vi "test.vi"() -> ()   [LabVIEW 2019]
uses:
  class/mqtt/mqttTypedef/mqttConnectionMeta.ctl
  class/mqtt/mqttTypedef/mqttQOSlevel.ctl
  class/mqtt/mqttTypedef/mqttSubscribeCluster.ctl
  class/mqtt/mqttTypedef/mqttConnectionStatus.ctl
  class/mqtt/mqttTXqueue/mqttTXdataQueueFunction.ctl
  class/mqtt/mqttConfigFunction.ctl
  class/mqtt/mqttTXqueue/mqttRXsubscriptionEventFunction.ctl
  class/mqtt/mqttTypedef/mqttBroker.ctl
  class/mqtt/mqttTypedef/mqttConnectionFlags.ctl
  class/mqtt/mqttTypedef/mqttWillInformation.ctl
  class/mqtt/mqtt.lvclass
panel:
  out "Ping Success":bool=TRUE
  in  "pingRequest":bool
  out "Numeric":i32
  out "messageID":u16
  out "RX Value":string
  out "RX Topic":string
  in  "includeTimeStamp":bool=TRUE
  in  "disconnect":bool
  out "sessionPresent":bool
  out "connStatus":T1
  in  "connect":bool
  in  "subscriptionInfo":T2[](array[typedef])=[{"Topic"="a/b", "QoS"=enum."At most once"}]
  out "subscribeMessageID":u16 format="%02x"
  out "subscribeSuccess":bool
  out "publishSuccess":bool=TRUE
  out "valueSent":string="14:19:17.238_"
  out "publishMessageID":u16 format="%02x"
  in  "connMeta":T4
  in  "value":string="abc"
  in  "topic":string="a/b"
  in  "quit":bool
  in  "subscribe":bool
  in  "publish":bool
  out "error out":errorcluster
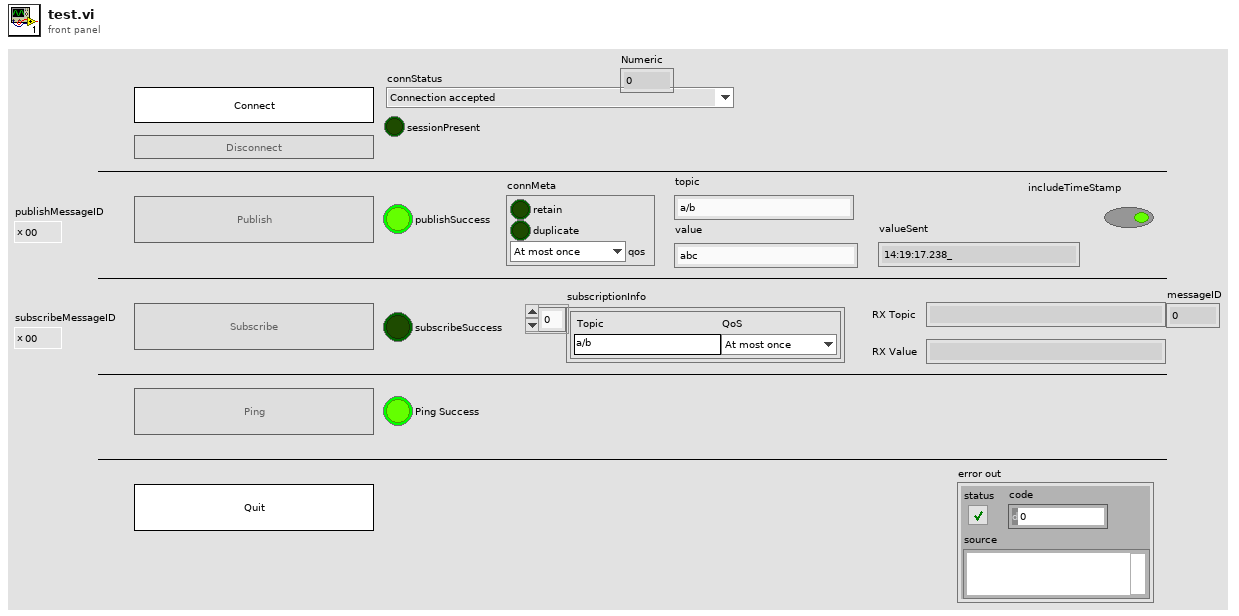
[diagram p1: front panel]
types:
  T1 = typedef "mqttConnectionStatus.ctl" = enum16{"Connection accepted", "Connection refused: unacceptable protocol version", "Connection refused: identifier rejected", "Connection refused: Server unavailable", "Connection refused: bad user name or password", "Connection refused: not authorized"}
  T2 = typedef "mqttSubscribeCluster.ctl" = cluster{"Topic":string, "QoS":T3}
  T3 = typedef "mqttQOSlevel.ctl" = enum8{"At most once", "At least once", "Exactly once", "Reserved"}
  T4 = typedef "mqttConnectionMeta.ctl" = cluster{"retain":bool, "duplicate":bool, "qos":T3}
  T5 = typedef "mqttWillInformation.ctl" = cluster{"User Name":string, "Password":string}
  T6 = typedef "mqttConnectionFlags.ctl" = cluster{"reserved":bool, "clean session":bool, "will flag":bool, "willQOS":enum8{"At most once", "At least once", "Exactly once", "Reserved"}, "will retain":bool, "password":bool, "user name":bool}
  T7 = typedef "mqttBroker.ctl" = cluster{"address":string, "port":u16, "connTimeout":i32, "writeTimeout":i32, "readTimeout":i32, "subTimeout":i32}
  T8 = typedef "mqttRXsubscriptionEventFunction.ctl" = enum16{"init", "deinit", "getEventRef", "event"}
  T9 = typedef "mqtt.lvclass/mqttConfigFunction.ctl" = enum16{"init", "deinit", "set", "get"}
  T10 = typedef "mqttTXdataQueueFunction.ctl" = enum16{"init", "deinit", "getQueue", "enqueue"}
  T11 = enum8{"Enabled", "Disabled", "Disabled and Grayed Out"}
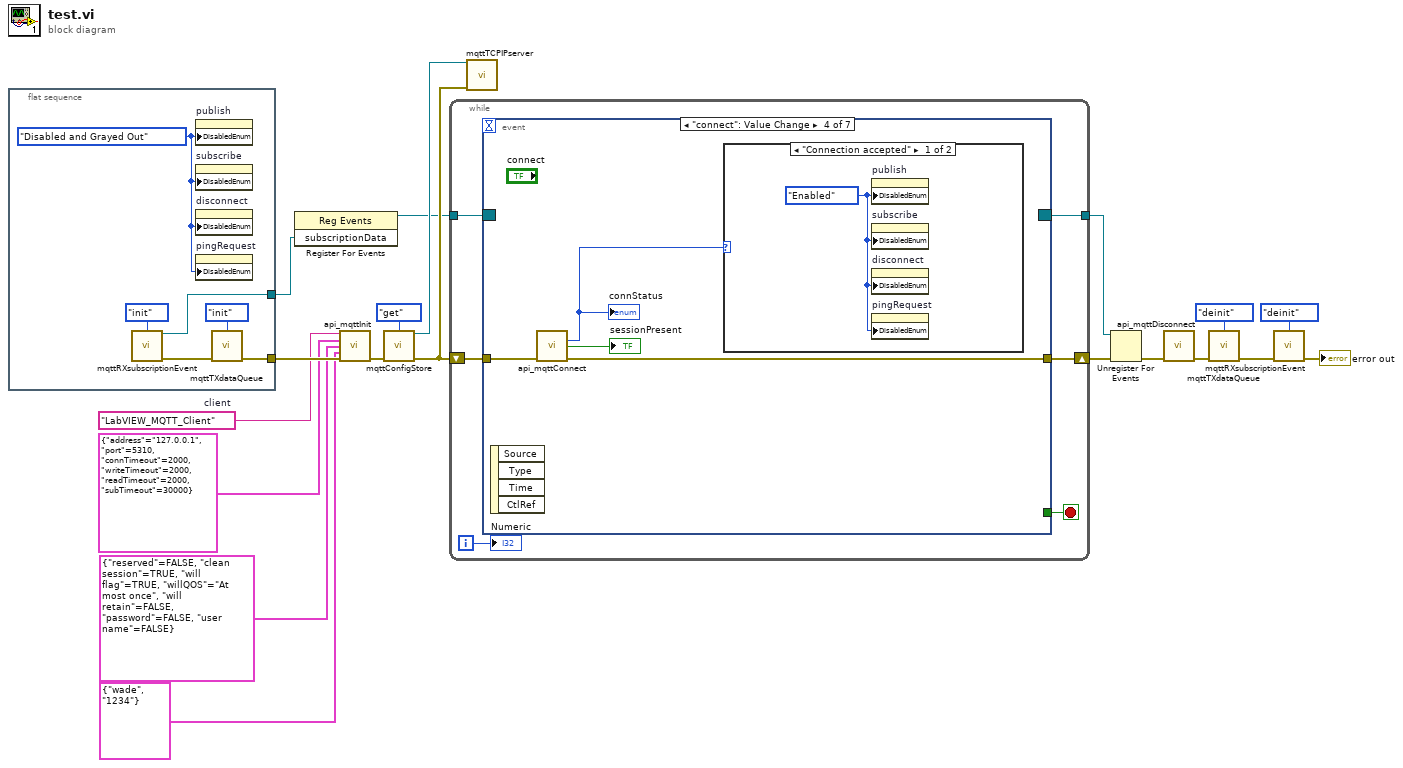
[diagram p0: block diagram]
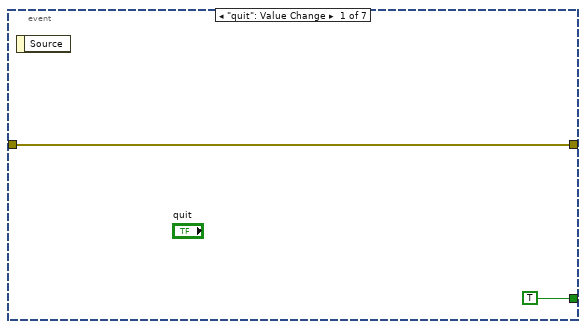
[diagram p2: hidden frame]
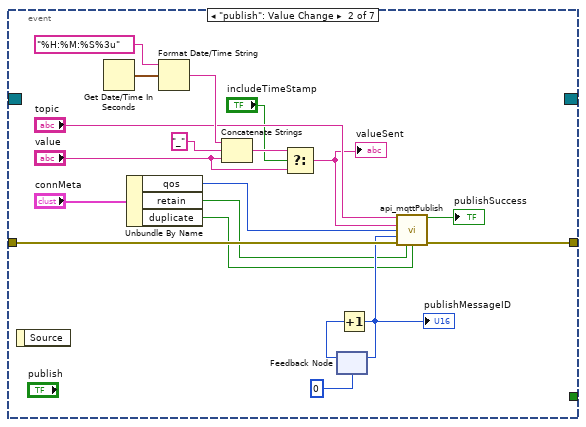
[diagram p3: hidden frame]
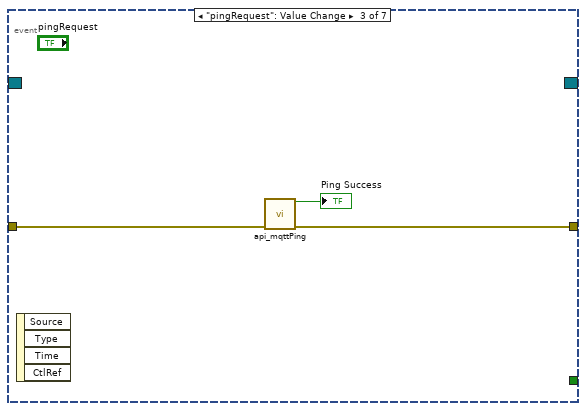
[diagram p4: hidden frame]
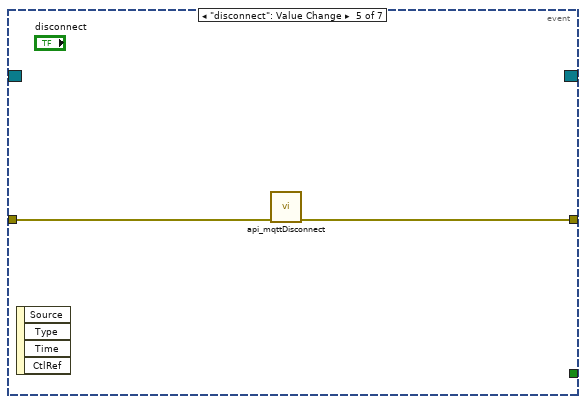
[diagram p6: hidden frame]
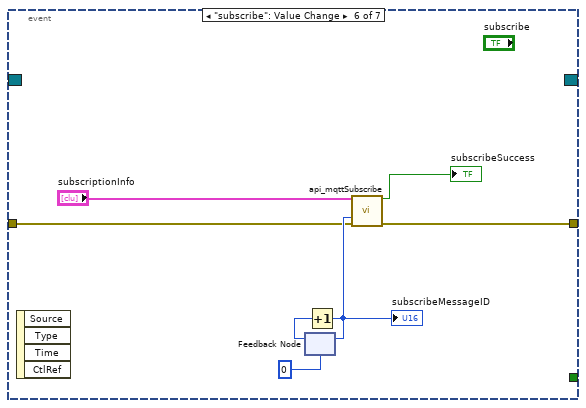
[diagram p7: hidden frame]
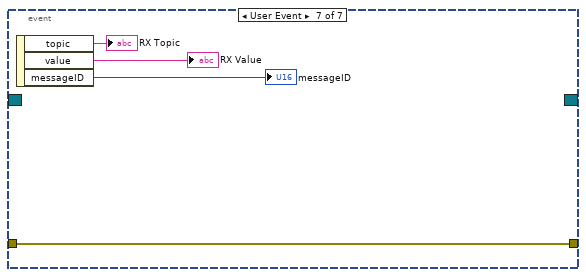
[diagram p8: hidden frame]
diagram:
  w4 = "LabVIEW_MQTT_Client"  # client
  n1 = flat-sequence {
    tunnel: [w24] -> w18
    tunnel: [w21] -> w12
    frame #0 {
      w20 = T11."Disabled and Grayed Out" ("Disabled")
      n2 = call "mqttRXsubscriptionEvent.vi"("function"=mqttRXsubscriptionEventFunction."init") -> ("subscriptionData"=w21:refnum<user-event>, "error out"=w23:errorcluster)  [unwired: 13 in]
      n3 = property on="publish" class="Bool"("DisabledEnum"=w20) -> ()  [unwired: 2 in, 2 out]
      n4 = property on="subscribe" class="Bool"("DisabledEnum"=w20) -> ()  [unwired: 2 in, 2 out]
      n5 = property on="disconnect" class="Bool"("DisabledEnum"=w20) -> ()  [unwired: 2 in, 2 out]
      n6 = property on="pingRequest" class="Bool"("DisabledEnum"=w20) -> ()  [unwired: 2 in, 2 out]
      n7 = call "mqttTXdataQueue.vi"("function"=mqttTXdataQueueFunction."init", "error in (no error)"=w23) -> ("error out"=w24:errorcluster)  [unwired: 12 in, 1 out]
    }
  }
  n8 = register-events(w12) -> (reference out=w11:refnum<event-registration>)  [unwired: 2 in, 1 out]
  n9 = call "api_mqttInit.vi"("client"=w4, "broker"=T7 {"address"="127.0.0.1", "port"=5310, "connTimeout"=2000, "writeTimeout"=2000, "readTimeout"=2000, "subTimeout"=30000}, "connFlags"=T6 {"reserved"=FALSE, "clean session"=TRUE, "will flag"=TRUE, "willQOS"=enum."At most once", "will retain"=FALSE, "password"=FALSE, "user name"=FALSE}, "User Info"=T5 {"User Name"="wade", "Password"="1234"}, "error in (no error)"=w18) -> ("error out"=w16:errorcluster)  [unwired: 10 in]
  n10 = call "mqttConfigStore.vi"("function"=mqttConfigFunction."get", "error in (no error)"=w16) -> ("mqtt.lvclass out"=w15:refnum<class "mqtt.lvclass">, "error out"=w14:errorcluster)  [unwired: 12 in]
  n11 = while {
    shift-right: [w31] -> w7
    shift-left: w14 -> [w30]
    tunnel: w11 -> [w28]
    tunnel: [w26] -> w5
    i -> [w27]
    stop <- w29 stop-if-true
    n12 = event shown="[3] \"connect\": Value Change" {
      selector: w28 -> [_ _ _ _ _ _ _]
      dyn-events: [_ _ _ _ _ _ _] -> w26
      timeout: _ -> [_ _ _ _ _ _ _]
      tunnel: [w32 w45 w54 w58 w61 w65 w73] -> w31
      tunnel: w30 -> [w32 w46 w55 w59 w62 w63 w73]
      tunnel: [TRUE _ _ _ _ _ _] -> w29
      event "quit": Value Change {
        n13 = event-data() -> ()  [unwired: 1 in, 1 out]
      }
      event "publish": Value Change {
        n14 = event-data() -> ()  [unwired: 1 in, 1 out]
        n15 = Get Date/Time In Seconds() -> (seconds since 1Jan1904=w52:timestamp)
        n16 = Unbundle By Name("connMeta") -> ("qos"=w40:T3, "retain"=w39:bool, "duplicate"=w38:bool)
        n17 = Format Date/Time String(time format string (%c)="%H:%M:%S%3u", seconds (now)=w52) -> (date/time string=w50:string)  [unwired: 1 in]
        n18 = Concatenate Strings(w50, "_", "value") -> (w37:string)
        n19 = Select(t=w37, s="includeTimeStamp", f="value") -> (s? t:f=w36:string)
        "valueSent" <- w36
        n20 = feedback #1(u16 0) -> (w47:u16)
        n21 = Increment(x=w47) -> (x+1=w44:u16)
        "publishMessageID" <- w44
        n22 = feedback-in #1(w44) -> ()
        n23 = call "api_mqttPublish.vi"("topic"="topic", "value"=w36, "QoS (At most once)"=w40, "messageID"=w44, "error in (no error)"=w46, "retain(F)"=w39, "duplicate(F)"=w38) -> ("success"=→"publishSuccess":bool, "error out"=w45:errorcluster)  [unwired: 7 in]
      }
      event "pingRequest": Value Change {
        n24 = event-data() -> ()  [unwired: 1 in, 4 out]
        n25 = call "api_mqttPing.vi"("error in (no error)"=w55) -> ("success"=→"Ping Success":bool, "error out"=w54:errorcluster)  [unwired: 13 in]
      }
      event "connect": Value Change {
        n26 = event-data() -> ()  [unwired: 1 in, 4 out]
        n27 = call "api_mqttConnect.vi"("error in (no error)"=w59) -> ("connStatus"=w56:T1, "sessionPresent"=→"sessionPresent":bool, "error out"=w58:errorcluster)  [unwired: 11 in, 1 out]
        "connStatus" <- w56
        n28 = case shown="\"Connection accepted\"" w56 {
          frame "Connection accepted" {
            w60 = T11."Enabled" ("Disabled")
            n29 = property on="publish" class="Bool"("DisabledEnum"=w60) -> ()  [unwired: 2 in, 2 out]
            n30 = property on="subscribe" class="Bool"("DisabledEnum"=w60) -> ()  [unwired: 2 in, 2 out]
            n31 = property on="disconnect" class="Bool"("DisabledEnum"=w60) -> ()  [unwired: 2 in, 2 out]
            n32 = property on="pingRequest" class="Bool"("DisabledEnum"=w60) -> ()  [unwired: 2 in, 2 out]
          }
          frame Default {
          }
        }
      }
      event "disconnect": Value Change {
        n33 = event-data() -> ()  [unwired: 1 in, 4 out]
        n34 = call "api_mqttDisconnect.vi"("error in (no error)"=w62) -> ("error out"=w61:errorcluster)  [unwired: 13 in, 1 out]
      }
      event "subscribe": Value Change {
        n35 = event-data() -> ()  [unwired: 1 in, 4 out]
        n36 = feedback #2(u16 0) -> (w68:u16)
        n37 = Increment(x=w68) -> (x+1=w64:u16)
        "subscribeMessageID" <- w64
        n38 = feedback-in #2(w64) -> ()
        n39 = call "api_mqttSubscribe.vi"("subscriptionInfo"="subscriptionInfo", "messageID"=w64, "error in (no error)"=w63) -> ("success"=→"subscribeSuccess":bool, "error out"=w65:errorcluster)  [unwired: 11 in]
      }
      event User Event {
        n40 = event-data() -> ("topic"=→"RX Topic":string, "value"=→"RX Value":string, "messageID"=→"messageID":u16)  [unwired: 1 in]
      }
    }
    "Numeric" <- w27
  }
  n41 = call "mqttTCPIPserver.vi"("mqtt.lvclass"=w15, "error in (no error)"=w14) -> ()  [unwired: 12 in, 2 out]
  n42 = Unregister For Events(event registration refnum=w5, error in=w7) -> (error out=w6:errorcluster)
  n43 = call "api_mqttDisconnect.vi"("error in (no error)"=w6) -> ("error out"=w13:errorcluster)  [unwired: 13 in, 1 out]
  n44 = call "mqttTXdataQueue.vi"("function"=mqttTXdataQueueFunction."deinit", "error in (no error)"=w13) -> ("error out"=w9:errorcluster)  [unwired: 12 in, 1 out]
  n45 = call "mqttRXsubscriptionEvent.vi"("function"=mqttRXsubscriptionEventFunction."deinit", "error in (no error)"=w9) -> ("error out"=→"error out":errorcluster)  [unwired: 12 in, 1 out]
